vi "KE2450_Meas_Resistance.vi"(4 "SENSE VLIM":dbl, 6 "Compliance Level (0.1)":dbl=0.1, 7 "Output Level (0)":dbl, 8 "error in (no error)":errorcluster, 9 "Enable Remote Sensing (T: Enable)":bool=TRUE, 10 "Source Mode  (0: Voltage)":u16(ring) items=["Voltage", "Current"], 11 "VISA resource name":refnum<visa-resource-name>) -> (0 "error out":errorcluster, 1 "Current Level Out (A)":dbl, 2 "Resistance (ohm)":dbl)   [LabVIEW 2017]
uses:
  Instrument Drivers/Keithley 2450/Keithley 2450.lvlib
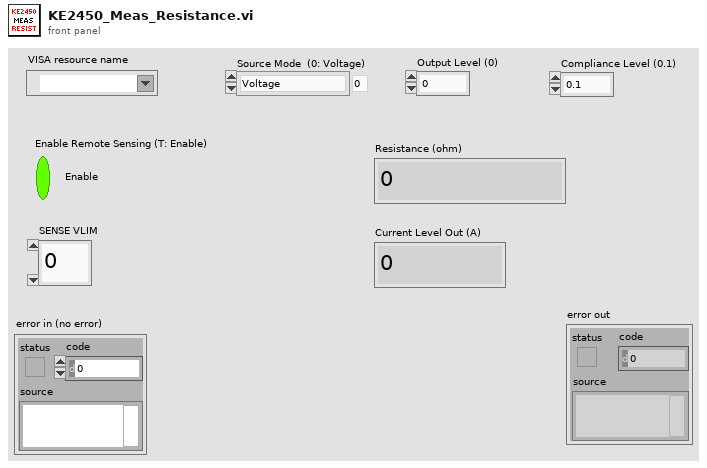
[diagram p1: front panel]
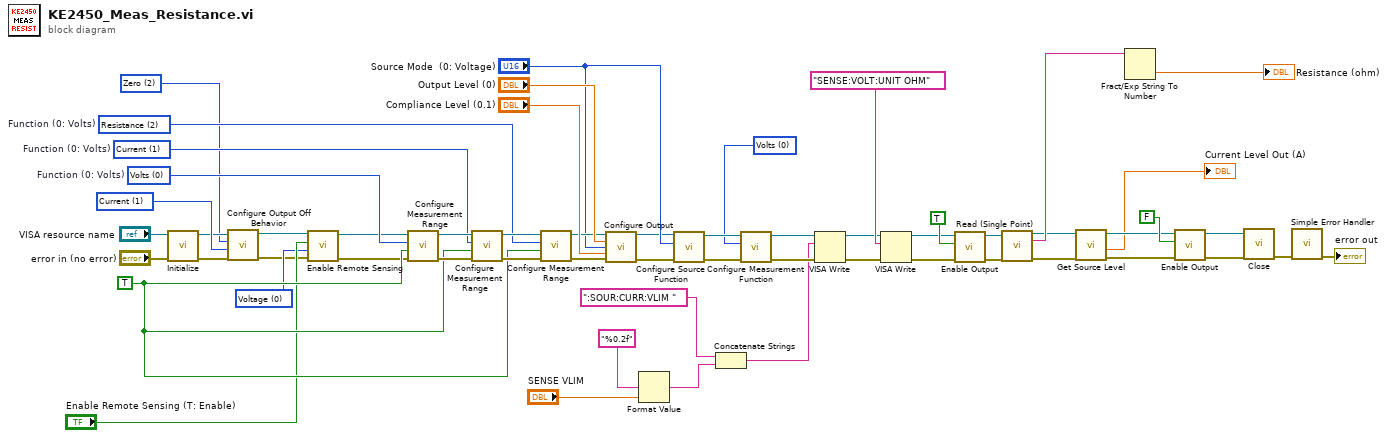
[diagram p0: block diagram]
diagram:
  w21 = u16 0 items=["Volts", "Current", "Auto Resistance", "Manual Resistance", "Digitize Voltage", "Digitize Current"] ("Function (0: Volts)")
  w27 = u16 2 items=["Normal", "High Impedance", "Zero", "Guard"] ("Output Off Behavior (0: Normal)")
  w29 = u16 1 items=["Volts", "Current"] ("Function (0: Volts)")
  w32 = u16 0 items=["Voltage", "Current", "Resistance", "Digitize Voltage", "Digitize Current"] ("Function (0:Voltage)")
  w36 = TRUE ("Enable Output (T: Enable)")
  w49 = u16 2 items=["Volts", "Current", "Resistance"]  # Function (0: Volts)
  w50 = u16 1 items=["Volts", "Current", "Resistance"]  # Function (0: Volts)
  w51 = u16 0 items=["Volts", "Current", "Resistance"]  # Function (0: Volts)
  n1 = call "Initialize.vi"("error in (no error)"="error in (no error)", "VISA resource name"="VISA resource name") -> ("error out"=w30:errorcluster, "VISA resource name out"=w28:refnum<visa-resource-name>)  [unwired: 8 in]
  n2 = call "Configure Output Off Behavior.vi"("error in (no error)"=w30, "Function (0: Volts)"=w29, "Output Off Behavior (0: Normal)"=w27, "VISA resource name"=w28) -> ("error out"=w25:errorcluster, "VISA resource name out"=w26:refnum<visa-resource-name>)  [unwired: 6 in]
  n3 = call "Enable Remote Sensing.vi"("error in (no error)"=w25, "Function (0:Voltage)"=w32, "Enable Remote Sensing (T: Enable)"="Enable Remote Sensing (T: Enable)", "VISA resource name"=w26) -> ("error out"=w34:errorcluster, "VISA resource name out"=w35:refnum<visa-resource-name>)  [unwired: 6 in]
  n4 = call "Configure Measurement Range.vi"("error in (no error)"=w34, "Enable Auto Range (T:Enable)"=w36, "Function (0: Volts)"=w51, "VISA resource name"=w35) -> ("error out"=w54:errorcluster, "VISA resource name out"=w55:refnum<visa-resource-name>)  [unwired: 6 in]
  n5 = call "Configure Measurement Range.vi"("error in (no error)"=w54, "Enable Auto Range (T:Enable)"=w36, "Function (0: Volts)"=w50, "VISA resource name"=w55) -> ("error out"=w53:errorcluster, "VISA resource name out"=w52:refnum<visa-resource-name>)  [unwired: 6 in]
  n6 = call "Configure Measurement Range.vi"("error in (no error)"=w53, "Enable Auto Range (T:Enable)"=w36, "Function (0: Volts)"=w49, "VISA resource name"=w52) -> ("error out"=w45:errorcluster, "VISA resource name out"=w44:refnum<visa-resource-name>)  [unwired: 6 in]
  n7 = call "Configure Output.vi"("VISA resource name"=w44, "Source Level (0)"="Output Level (0)", "Source Mode  (0: Voltage)"="Source Mode  (0: Voltage)", "Source Limit Level (0.1)"="Compliance Level (0.1)", "error in (no error)"=w45) -> ("VISA resource name out"=w11:refnum<visa-resource-name>, "error out"=w10:errorcluster)  [unwired: 9 in]
  n8 = Format Value(format string="%0.2f" ("string (\"\")"), value (0)="SENSE VLIM") -> (output string=w4:string)  [unwired: 1 in]
  n9 = call "Configure Source Function.vi"("error in (no error)"=w10, "Function (0: Volts)"="Source Mode  (0: Voltage)", "VISA resource name"=w11) -> ("error out"=w39:errorcluster, "VISA resource name out"=w38:refnum<visa-resource-name>)  [unwired: 7 in]
  n10 = Concatenate Strings(":SOUR:CURR:VLIM " ("write buffer"), w4) -> (w2:string)
  n11 = call "Configure Measurement Function.vi"("error in (no error)"=w39, "Function (0: Volts)"=w21, "VISA resource name"=w38) -> ("error out"=w9:errorcluster, "VISA resource name out"=w7:refnum<visa-resource-name>)  [unwired: 7 in]
  n12 = VISA Write(VISA resource name=w7, write buffer=w2, error in (no error)=w9) -> (VISA resource name out=w6:refnum<visa-resource-name>, error out=w8:errorcluster)  [unwired: 1 out]
  n13 = VISA Write(VISA resource name=w6, write buffer="SENSE:VOLT:UNIT OHM", error in (no error)=w8) -> (VISA resource name out=w15:refnum<visa-resource-name>, error out=w14:errorcluster)  [unwired: 1 out]
  n14 = call "Enable Output.vi"("error in (no error)"=w14, "Enable Output (T: Enable)"=TRUE, "VISA resource name"=w15) -> ("error out"=w23:errorcluster, "VISA resource name out"=w22:refnum<visa-resource-name>)  [unwired: 7 in]
  n15 = call "Read (Single Point).vi"("VISA resource name"=w22, "error in (no error)"=w23) -> ("VISA resource name out"=w20:refnum<visa-resource-name>, "Data out"=w40:string, "error out"=w19:errorcluster)  [unwired: 11 in]
  n16 = call "Get Source Level.vi"("error in (no error)"=w19, "VISA resource name"=w20) -> ("error out"=w18:errorcluster, "Current Level Out"=→"Current Level Out (A)":dbl, "VISA resource name out"=w17:refnum<visa-resource-name>)  [unwired: 6 in, 1 out]
  n17 = Fract/Exp String To Number(string=w40) -> (number=→"Resistance (ohm)":dbl)  [unwired: 3 in, 1 out]
  n18 = call "Enable Output.vi"("error in (no error)"=w18, "Enable Output (T: Enable)"=FALSE, "VISA resource name"=w17) -> ("error out"=w41:errorcluster, "VISA resource name out"=w42:refnum<visa-resource-name>)  [unwired: 7 in]
  n19 = call "Close.vi"("error in (no error)"=w41, "VISA resource name"=w42) -> ("error out"=w57:errorcluster)  [unwired: 9 in]
  n20 = call <vilib>:"Simple Error Handler.vi"("error in (no error)"=w57) -> ("error out"=→"error out":errorcluster)  [unwired: 4 in, 4 out]
